vi "SCP Close.vi"(8 "Error In":errorcluster, 11 "SCP Session":refnum<k24>) -> (0 "Error Out":errorcluster)   [LabVIEW 2024, in "LMH-LINX.lvlib"]
uses:
  <vilib>/MakerHub/LINX/LMH-LINX.lvlib
  <vilib>/MakerHub/LINX/Resources/Renci.SshNet.dll
  <vilib>/net/SFTP/Session/Session.lvclass
  <vilib>/MakerHub/LINX/Private/Utilties/SSH/SSH OpenSSH Session Op.ctl
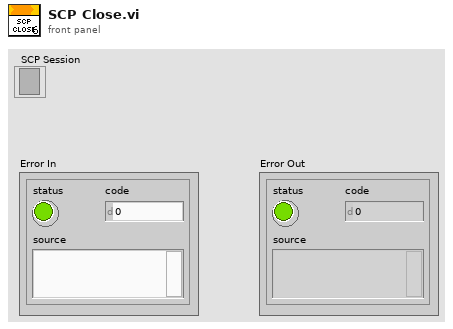
[diagram p1: front panel]
types:
  T1 = typedef "LMH-LINX.lvlib/SSH OpenSSH Session Op.ctl" = enum16{"Get", "Set"}
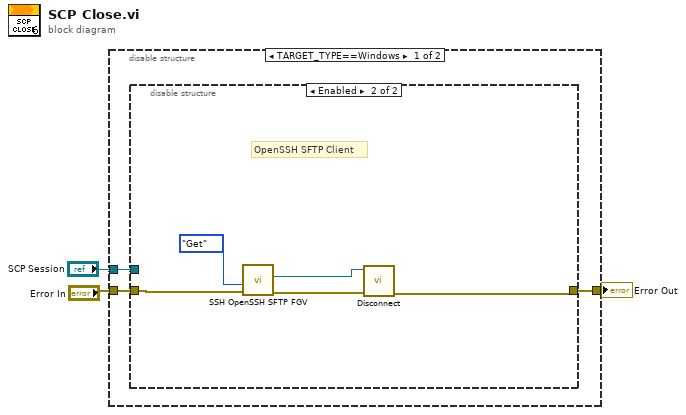
[diagram p0: block diagram]
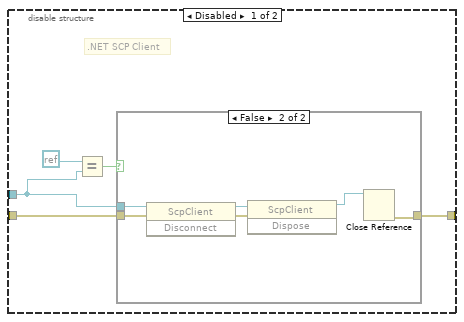
[diagram p2: hidden frame]
diagram:
  n1 = disable-structure shown="TARGET_TYPE==Windows" {
    disable-tunnel: [w6 w24] -> w3
    disable-tunnel: "Error In" -> [w5 w24]
    disable-tunnel: "SCP Session" -> [w4 _]
    frame condition #0 (active) {
      n2 = disable-structure shown="Enabled" {
        disable-tunnel: [w11 w23] -> w6
        disable-tunnel: w5 -> [w10 w21]
        disable-tunnel: w4 -> [w8 _]
        frame Disabled {
          # ".NET SCP Client"
          n3 = Equal?(x=refnum<k0> refnum, y=w8) -> (x = y?=w7:bool)
          n4 = case shown="False" w7 {
            tunnel: [w12 w13] -> w11
            tunnel: w10 -> [w12 w16]
            tunnel: w8 -> [_ w15]
            frame True {
            }
            frame False {
              n5 = invoke class="ScpClient" method="Disconnect"(reference=w15, error in=w16) -> (reference out=w18:refnum<k24>, error out=w17:errorcluster)  [unwired: 1 in, 1 out]
              n6 = invoke class="ScpClient" method="Dispose"(reference=w18, error in=w17) -> (reference out=w14:refnum<k24>)  [unwired: 1 in, 2 out]
              n7 = Close Reference(reference=w14) -> (error out=w13:errorcluster)  [unwired: 1 in]
            }
          }
        }
        frame Enabled {
          # "OpenSSH SFTP Client"
          n8 = call <vilib>:"SSH OpenSSH SFTP FGV.vi"("error in (no error)"=w21, "OpenSSH Session Op"=SSH_OpenSSH_Session_Op."Get") -> ("error out"=w20:errorcluster, "OpenSSH Session out"=w19:refnum<class "Session.lvclass">)  [unwired: 7 in, 1 out]
          n9 = call-dynamic "Disconnect.vi"("error in"=w20, "session in"=w19) -> ("error out"=w23:errorcluster)  [unwired: 6 in, 3 out]
        }
      }
    }
    frame condition #1 {
    }
  }
  "Error Out" <- w3
